vi "GVSDataView Mark Window Right.vi"() -> ()   [LabVIEW 2013]
uses:
  <vilib>/Utility/miscctls.llb/LVPositionTypeDef.ctl
  SubVI/GVSMain Sub Window Global.vi
  GVSNew View Global.vi
panel:
  in  "sMe":string
  in  "bShow":bool=TRUE
  in  "Right":bool
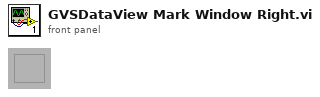
[diagram p1: front panel]
types:
  T1 = typedef "LVPositionTypeDef.ctl" = cluster{"Left":i32, "Top":i32}
  T2 = typedef "LVRectTypeDef.ctl" = cluster{"Left":i16, "Top":i16, "Right":i16, "Bottom":i16}
  T3 = typedef "Graph Main Info Cluster.ctl" = cluster{"Selected_BarIdx":i32, "Selected_PanelIdx":i32, "Graph Main VIRef":refnum<vi>, "ToolBarClick":bool, "Spliter Ref Array":refnum<vi>[], "Panel Ref Array":refnum<vi>[], "Spliter_matrix":i32[][], "Panel_matrix":i32[][], "child_spliterIdx_matrix":i32[][], "split_pos_matrix":i32[][], "Title State":bool, "sQueueName":string, "Frame nID":i32, "Graph VIRef Array":cluster{"Graph VIRef":refnum<vi>, "Panel Idx":i32, "Frame VIRef":refnum<vi>, "Icon Ring":i32, "Graph Type":string}[], "View Type":string}
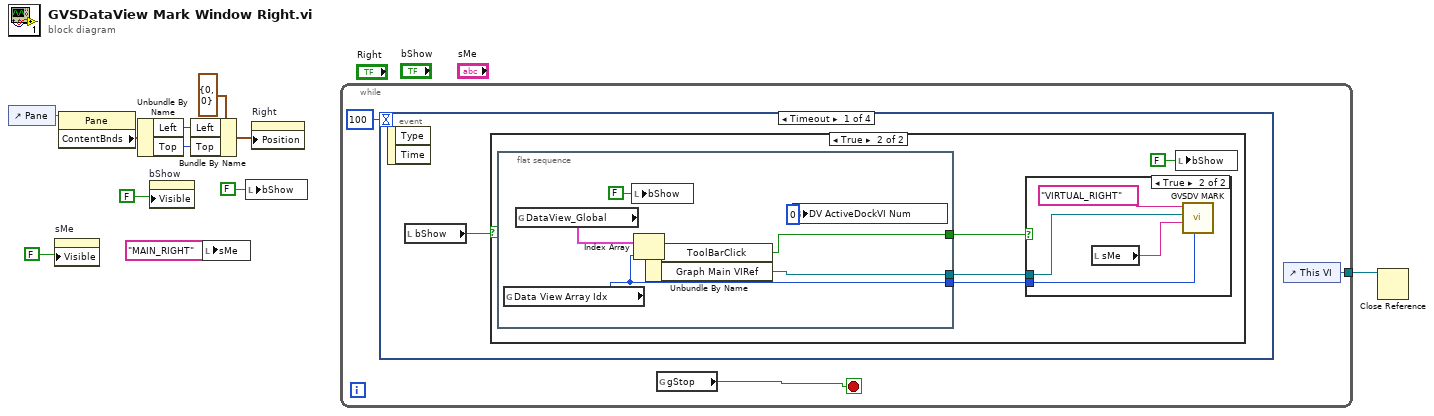
[diagram p0: block diagram]
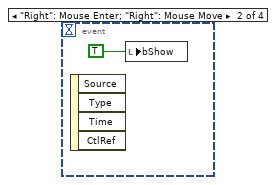
[diagram p4: hidden frame]
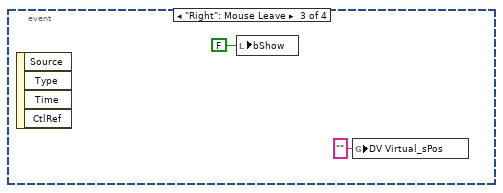
[diagram p5: hidden frame]
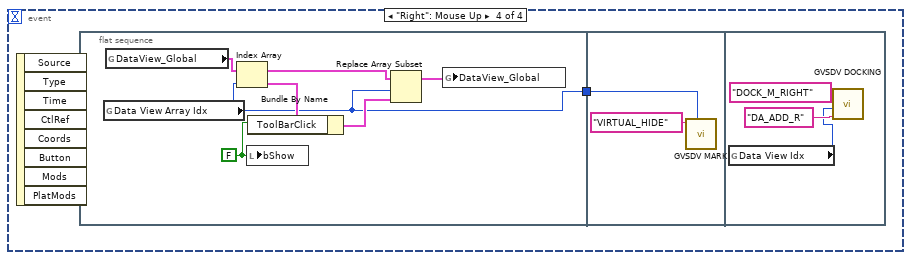
[diagram p6: hidden frame]
diagram:
  n1 = control-ref of="Pane"() -> (w11:refnum<vi>)
  n2 = property on="sMe" class="Str"("Visible"=FALSE) -> ()  [unwired: 2 in, 2 out]
  n3 = property class="Pane"(reference=w11) -> ("ContentBnds"=w10:T2)  [unwired: 1 in, 2 out]
  n4 = Unbundle By Name(w10) -> ("Left"=w9:i16, "Top"=w7:i16)
  n5 = property on="bShow" class="Bool (strict)"("Visible"=FALSE) -> ()  [unwired: 2 in, 2 out]
  n6 = Bundle By Name(cluster=T1 {"Left"=0, "Top"=0} ("Position"), "Left"=w9, "Top"=w7) -> (w6:T1)
  n7 = local write "sMe"("MAIN_RIGHT" ("sMe")) -> ()
  n8 = local write "bShow"(FALSE ("bShow")) -> ()
  n9 = property on="Right" class="Bool (strict)"("Position"=w6) -> ()  [unwired: 2 in, 2 out]
  n10 = while {
    tunnel: [w13] -> w1
    stop <- w12 stop-if-true
    n11 = event shown="[0] Timeout" {
      selector: _ -> [_ _ _ _]
      dyn-events: _ -> [_ _ _ _]
      timeout: 100 -> [_ _ _ _]
      event Timeout {
        n12 = event-data() -> ()  [unwired: 3 out]
        n13 = local read "bShow"() -> (w15:bool)
        n14 = case shown="True" w15 {
          frame False {
          }
          frame True {
            n15 = flat-sequence {
              tunnel: [w25] -> w18
              tunnel: [w23] -> w17
              tunnel: [w22] -> w16
              frame #0 {
                n16 = global read "GVSNew View Global.vi" "Data View Array Idx"() -> (w22:i32)
                n17 = global read "GVSNew View Global.vi" "DataView_Global"() -> (w21:T3[])
                n18 = local write "bShow"(FALSE ("bShow")) -> ()
                n19 = Index Array(array=w21, index=w22) -> (element=w26:T3)
                n20 = Unbundle By Name(w26) -> ("ToolBarClick"=w25:bool, "Graph Main VIRef"=w23:refnum<vi>)
                n21 = global write "GVSNew View Global.vi" "DV ActiveDockVI Num"(0 ("ActiveDockVI Num")) -> ()
              }
            }
            n22 = case shown="True" w18 {
              tunnel: w17 -> [_ w29]
              tunnel: w16 -> [_ w27]
              frame False {
              }
              frame True {
                n23 = local read "sMe"() -> (w28:string)
                n24 = call "GVSDV MARK.vi"("sAction"="VIRTUAL_RIGHT", "mVritual_VIRef"=w29, "sData"=w28, "DataView Array Index"=w27) -> ()  [unwired: 6 in, 1 out]
              }
            }
            n25 = local write "bShow"(FALSE ("bShow")) -> ()
          }
        }
      }
      event "Right": Mouse Enter; "Right": Mouse Move {
        n26 = event-data() -> ()  [unwired: 5 out]
        n27 = local write "bShow"(TRUE ("bShow")) -> ()
      }
      event "Right": Mouse Leave {
        n28 = event-data() -> ()  [unwired: 5 out]
        n29 = local write "bShow"(FALSE ("bShow")) -> ()
        n30 = global write "GVSNew View Global.vi" "DV Virtual_sPos"("" ("DV Virtual_sPos")) -> ()
      }
      event "Right": Mouse Up {
        n31 = event-data() -> ()  [unwired: 9 out]
        n32 = flat-sequence {
          tunnel: [w37] -> w34
          tunnel: w34 -> [w41]
          frame #0 {
            w38 = FALSE ("bShow")
            n33 = global read "GVSNew View Global.vi" "Data View Array Idx"() -> (w37:i32)
            n34 = global read "GVSNew View Global.vi" "DataView_Global"() -> (w36:T3[])
            n35 = Index Array(array=w36, index=w37) -> (element=w39:T3)
            n36 = local write "bShow"(w38) -> ()
            n37 = Bundle By Name(cluster=w39, "ToolBarClick"=w38) -> (w40:T3)
            n38 = Replace Array Subset(array=w36, new element=w40, index=w37) -> (w35:T3[])
            n39 = global write "GVSNew View Global.vi" "DataView_Global"(w35) -> ()
          }
          frame #1 {
            n40 = call "GVSDV MARK.vi"("sAction"="VIRTUAL_HIDE", "DataView Array Index"=w41) -> ()  [unwired: 8 in, 1 out]
          }
          frame #2 {
            n41 = global read "GVSNew View Global.vi" "Data View Idx"() -> (w43:i32)
            n42 = call "GVSDV DOCKING.vi"("sData"="DA_ADD_R" ("Action Type"), "DataView Index"=w43, "sAction"="DOCK_M_RIGHT") -> ()  [unwired: 5 in, 4 out]
          }
        }
      }
    }
    n43 = global read "GVSMain Sub Window Global.vi" "gStop"() -> (w12:bool)
    n44 = control-ref of="This VI"() -> (w13:refnum<vi>)
  }
  n45 = Close Reference(reference=w1) -> ()  [unwired: 1 in, 1 out]
